vi "New from bool.vi"(8 "error in (no error)":errorcluster) -> (0 "error out":errorcluster, 2 "MsgPackBool out":refnum<class "MsgPackBool.lvclass">)   [LabVIEW 2020, in "MessagePack.lvlib" / "MsgPackBool.lvclass"]
uses:
  MsgPackBool.lvclass
  MsgPackBool.lvclass/MsgPackBool.ctl
panel:
  in  "Boolean in":bool
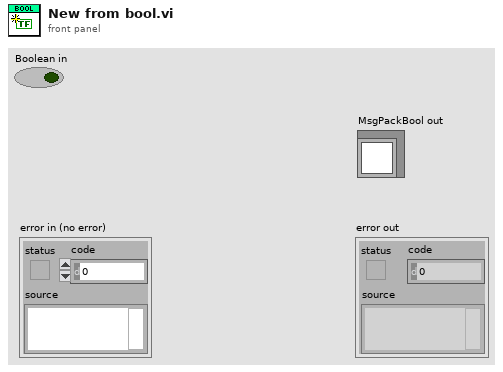
[diagram p1: front panel]
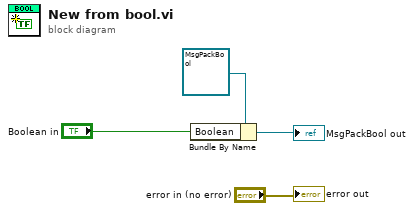
[diagram p0: block diagram]
diagram:
  n1 = Bundle By Name(cluster=refnum<class "MsgPackBool.lvclass"> refnum ("MessagePack.lvlib:MsgPackBool.lvclass"), "Boolean"="Boolean in") -> (→"MsgPackBool out":refnum<class "MsgPackBool.lvclass">)
  "error out" <- "error in (no error)"
